vi "MC - Test Interval String.vi"(0 "interval string":string) -> (1 "valid interval":bool, 2 "interval string is \"interval\"":bool)   [LabVIEW 2015]
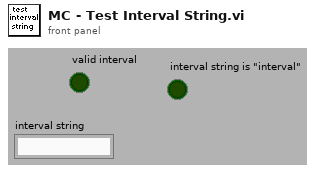
[diagram p1: front panel]
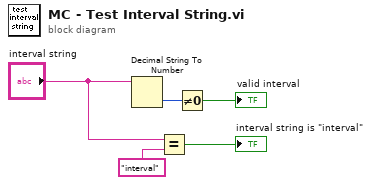
[diagram p0: block diagram]
diagram:
  n1 = Decimal String To Number(string="interval string") -> (number=w5:i32)  [unwired: 3 out]
  n2 = Equal?(x="interval string", y="interval") -> (x = y?=→"interval string is \"interval\"":bool)
  n3 = Not Equal To 0?(x=w5) -> (x != 0?=→"valid interval":bool)
